vi "InterpRoute.vi"(8 "error in (no error)":errorcluster, 10 "GridSize(mm)":dbl=1.0 format="%#_13g", 11 "FollowScanWOffset":cluster{"x(mm)":dbl, "y(mm)":dbl, "z(mm)":dbl}[](array[cluster])) -> (0 "error out":errorcluster, 1 "Zi":dbl[](array[numeric]), 2 "Yi":dbl[](array[numeric]), 3 "Xi":dbl[](array[numeric]), 4 "Dim out":cluster{"X":i32, "Y":i32})   [LabVIEW 2024]
uses:
  <vilib>/gmath/interp.llb/Interpolate 2D Scattered (1D).vi
  <vilib>/gmath/NI_AAL_Interpolation.lvlib
panel:
  out "Waveform Graph":dbl[](graph)
  out "Y":dbl[](array[numeric])
  out "X":dbl[](array[numeric])
  out "Z":dbl[](array[numeric])
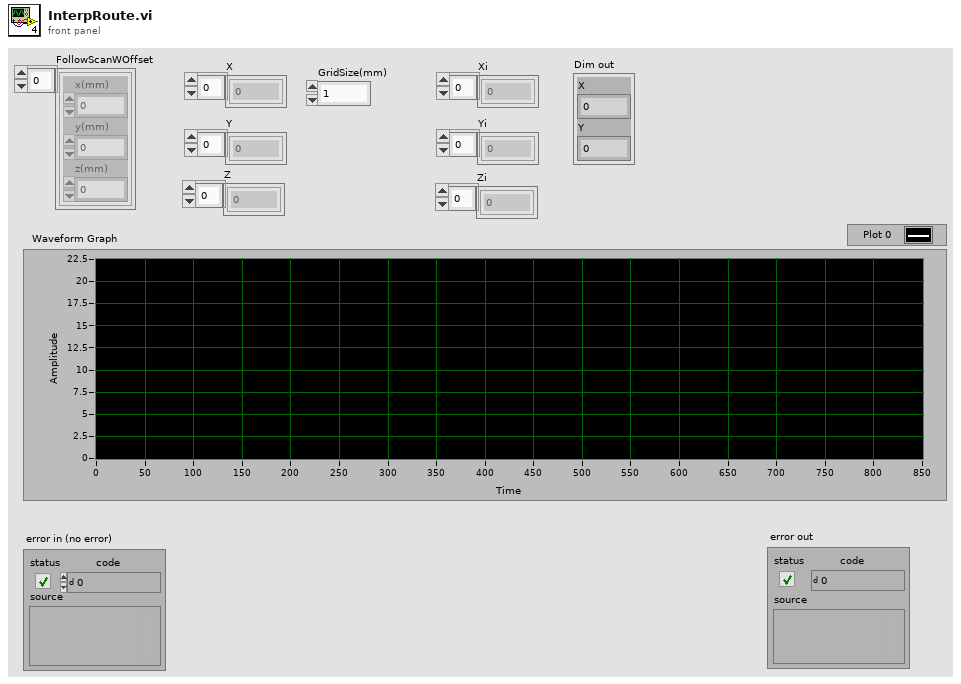
[diagram p1: front panel]
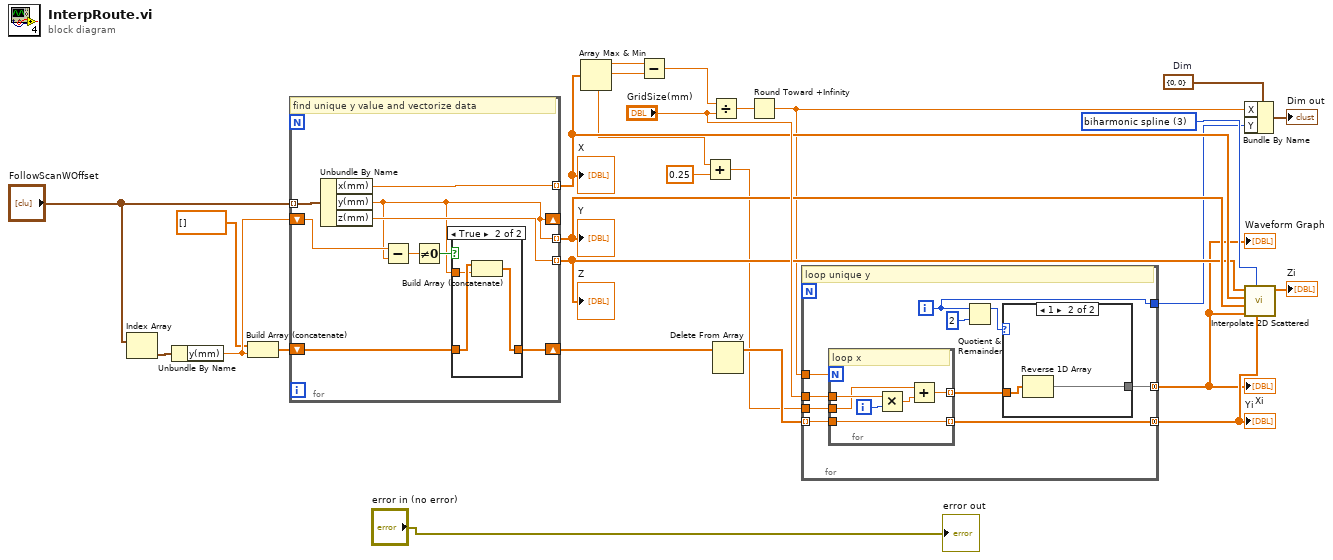
[diagram p0: block diagram]
diagram:
  w13 = cluster{"X":i32, "Y":i32} {"X"=0, "Y"=0}  # Dim
  w20 = 3 items=["nearest", "linear", "cubic", "biharmonic spline "] ("method")
  n1 = Index Array(array="FollowScanWOffset") -> (element=w6:cluster{"x(mm)":dbl, "y(mm)":dbl, "z(mm)":dbl})  [unwired: 1 in]
  n2 = Unbundle By Name(w6) -> ("y(mm)"=w9:dbl)
  n3 = Build Array (concatenate)(dbl[] [], w9) -> (w8:dbl[])
  n4 = for {
    tunnel: [w31] -> w18 mode=indexing
    shift-right: [w27] -> _
    shift-left: w9 -> [w30]
    shift-right: [w33] -> w21
    shift-left: w8 -> [w32]
    tunnel: "FollowScanWOffset" -> [w29] mode=indexing
    tunnel: [w28] -> w17 mode=indexing
    tunnel: [w27] -> w19 mode=indexing
    # "find unique y value and vectorize data"
    n5 = Unbundle By Name(w29) -> ("x(mm)"=w31:dbl, "y(mm)"=w27:dbl, "z(mm)"=w28:dbl)
    n6 = Subtract(x=w30, y=w27) -> (x-y=w35:dbl)
    n7 = Not Equal To 0?(x=w35) -> (x != 0?=w34:bool)
    n8 = case shown="True" w34 {
      tunnel: [w36 w39] -> w33
      tunnel: w32 -> [w36 w38]
      tunnel: w27 -> [_ w37]
      frame False {
      }
      frame True {
        n9 = Build Array (concatenate)(w38, w37) -> (w39:dbl[])
      }
    }
  }
  "Z" <- w17
  "X" <- w18
  "Y" <- w19
  n10 = Array Max & Min(array=w18) -> (max value=w24:dbl, min value=w4:dbl)  [unwired: 2 out]
  n11 = Subtract(x=w24, y=w4) -> (x-y=w15:dbl)
  n12 = Add(x=w4, y=0.25) -> (x+y=w2:dbl)
  n13 = Divide(x=w15, y="GridSize(mm)") -> (x/y=w16:dbl)
  n14 = Delete From Array(array=w21) -> (array with subset deleted=w22:dbl[])  [unwired: 2 in, 1 out]
  n15 = Round Toward +Infinity(x=w16) -> (ceil(x): smallest int >= x=w12:dbl)
  n16 = for {
    tunnel: w12 -> [w49]
    tunnel: "GridSize(mm)" -> [w48]
    tunnel: w2 -> [w47]
    tunnel: w22 -> [w46] mode=indexing
    tunnel: [w45] -> w25 mode=concatenating
    tunnel: [w41] -> w5 mode=concatenating
    tunnel: [w40] -> w11
    i -> [w40]
    # "loop unique y"
    n17 = for {
      N: w49 -> [_]
      tunnel: w48 -> [w57]
      tunnel: w47 -> [w55]
      tunnel: [w54] -> w42 mode=indexing
      tunnel: [w53] -> w45 mode=indexing
      tunnel: w46 -> [w53]
      i -> [w58]
      # "loop x"
      n18 = Multiply(x=w57, y=w58) -> (x*y=w56:dbl)
      n19 = Add(x=w55, y=w56) -> (x+y=w54:dbl)
    }
    n20 = Quotient & Remainder(x=w40, y=2) -> (x-y*floor(x/y)=w43:i32)  [unwired: 1 out]
    n21 = case shown="1" w43 {
      tunnel: w42 -> [w50 w52]
      tunnel: [w50 w51] -> w41
      frame 0, Default {
      }
      frame 1 {
        n22 = Reverse 1D Array(array=w52) -> (reversed array=w51:dbl[])
      }
    }
  }
  "Yi" <- w25
  "Xi" <- w5
  "Waveform Graph" <- w5
  n23 = Bundle By Name(cluster=w13, "X"=w12, "Y"=w11) -> (→"Dim out":cluster{"X":i32, "Y":i32})
  n24 = call-poly <vilib>:"Interpolate 2D Scattered.vi"("Yi"=w25, "method"=w20, "Xi"=w5, "Y"=w19, "X"=w18, "Z"=w17) -> ("Zi"=→"Zi":dbl[])  [unwired: 4 in, 1 out]
  "error out" <- "error in (no error)"
